vi "Decode Cluster.vi"(9 "Input Value":variant, 10 "Controls Refs[]":refnum<vi>[](array[refnum]), 11 "Cluster Name":string) -> (0 "error out":errorcluster, 1 "Cluster Component Values":variant[](array[variant]), 2 "Cluster Component Names":string[](array[string]), 3 "Cluster Refnum":refnum<vi>, 5 "Cluster Size":i32)   [LabVIEW 2021]
panel:
  out "Found?":bool
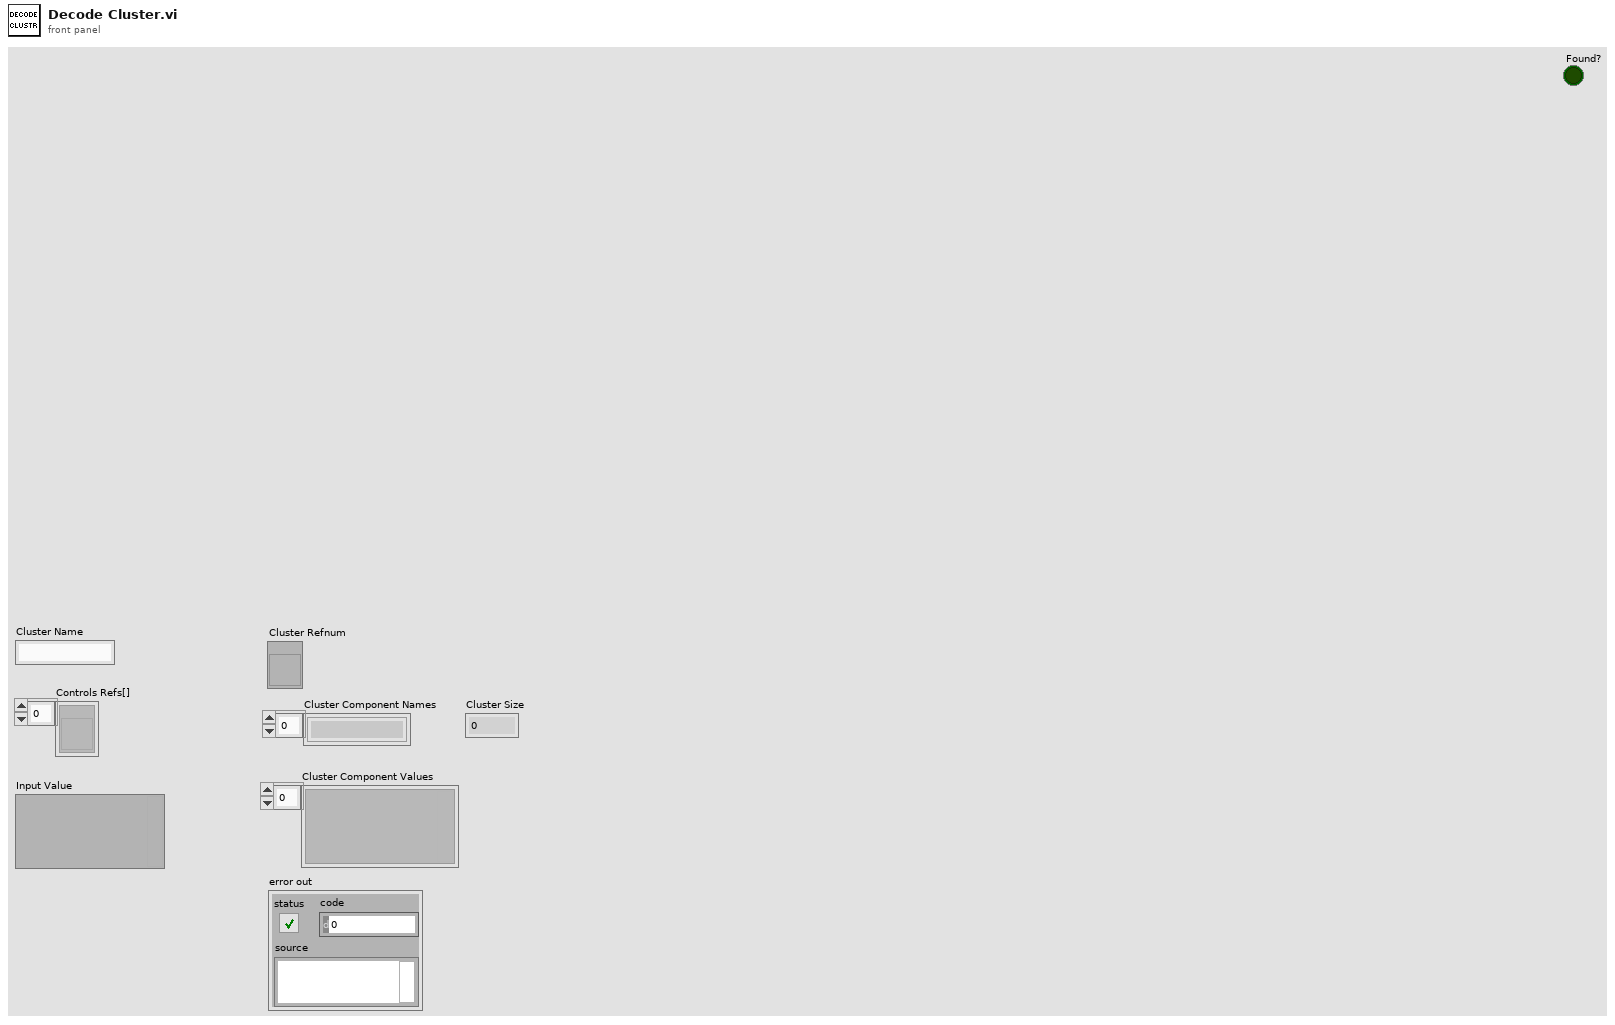
[diagram p1: front panel]
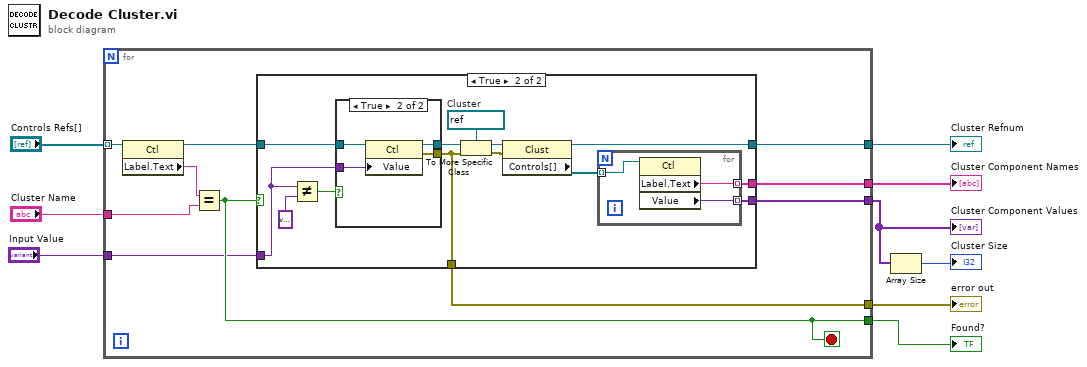
[diagram p0: block diagram]
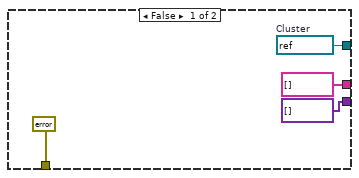
[diagram p2: hidden frame]
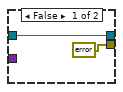
[diagram p3: hidden frame]
diagram:
  n1 = for {
    tunnel: "Controls Refs[]" -> [w19] mode=indexing
    tunnel: "Cluster Name" -> [w18]
    tunnel: [w16] -> w9
    tunnel: "Input Value" -> [w15]
    tunnel: [w13] -> w5
    tunnel: [w12] -> w4
    tunnel: [w11] -> w2
    tunnel: [w10] -> w1
    stop <- w16 stop-if-true
    n2 = property class="Ctl"(reference=w19) -> (reference out=w14:refnum<vi>, "Label.Text"=w17:string)  [unwired: 1 in, 1 out]
    n3 = Equal?(x=w17, y=w18) -> (x = y?=w16:bool)
    n4 = case shown="True" w16 {
      tunnel: w15 -> [_ w33]
      tunnel: w14 -> [_ w32]
      tunnel: [w23 w27] -> w13
      tunnel: [string[] [] w26] -> w12
      tunnel: [variant[] [] w25] -> w11
      tunnel: [errorcluster {"status"=FALSE, "code"=0, "source"=""} ("error out") w24] -> w10
      frame False {
        w23 = refnum<vi> refnum  # Cluster
      }
      frame True {
        w28 = refnum<vi> refnum  # Cluster
        n5 = Not Equal?(x=w33, y=variant ("x")) -> (x != y?=w36:bool)
        n6 = case shown="True" w36 {
          tunnel: [w38 w42] -> w30
          tunnel: w33 -> [_ w41]
          tunnel: w32 -> [w38 w40]
          tunnel: [errorcluster {"status"=FALSE, "code"=0, "source"=""} ("error out") w39] -> w24
          frame False {
          }
          frame True {
            n7 = property class="Ctl"(reference=w40, "Value"=w41) -> (reference out=w42:refnum<vi>, error out=w39:errorcluster)  [unwired: 1 in]
          }
        }
        n8 = To More Specific Class(target class=w28, reference=w30, error in=w24) -> (specific class reference=w29:refnum<vi>, error out=w31:errorcluster)
        n9 = property class="Clust"(reference=w29, error in=w31) -> (reference out=w27:refnum<vi>, "Controls[]"=w35:refnum<vi>[])  [unwired: 1 out]
        n10 = for {
          tunnel: w35 -> [w45] mode=indexing
          tunnel: [w44] -> w26 mode=indexing
          tunnel: [w43] -> w25 mode=indexing
          n11 = property class="Ctl"(reference=w45) -> ("Label.Text"=w44:string, "Value"=w43:variant)  [unwired: 1 in, 2 out]
        }
      }
    }
  }
  "Cluster Component Names" <- w4
  "Cluster Component Values" <- w2
  "Found?" <- w9
  "Cluster Refnum" <- w5
  "error out" <- w1
  n12 = Array Size(array=w2) -> (size(s)=→"Cluster Size":i32)
